vi "kDelay.vi"(8 "delay":i32=10, 11 "input":dbl) -> (3 "output":dbl)   [LabVIEW 2016, in "kevLib2010.lvlib"]
uses:
  kevLib2010.lvlib
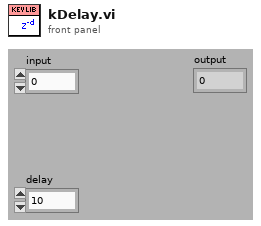
[diagram p1: front panel]
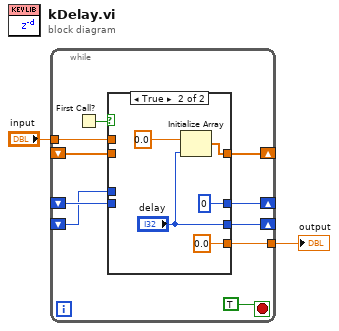
[diagram p0: block diagram]
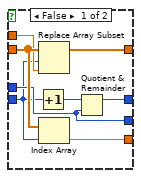
[diagram p2: hidden frame]
diagram:
  n1 = while {
    shift-right: [w11] -> _
    shift-left: _ -> [w10]
    shift-right: [w9] -> _
    shift-left: _ -> [w8]
    shift-right: [w7] -> _
    shift-left: _ -> [w6]
    tunnel: "input" -> [w5]
    tunnel: [w3] -> w1
    stop <- TRUE stop-if-true
    n2 = First Call?() -> (First Call?: T/F=w12:bool)
    n3 = case shown="True" w12 {
      tunnel: [w19 w25] -> w11
      tunnel: w10 -> [w20 _]
      tunnel: [w16 0 ("index")] -> w9
      tunnel: w8 -> [w14 _]
      tunnel: [w17 "delay"] -> w7
      tunnel: w6 -> [w17 _]
      tunnel: w5 -> [w15 _]
      tunnel: [w13 0.0 ("input")] -> w3
      frame False {
        n4 = Increment(x=w14) -> (x+1=w18:i32)
        n5 = Replace Array Subset(array=w20, new element=w15, index=w14) -> (w19:dbl[])
        n6 = Index Array(array=w20, index=w14) -> (element=w13:dbl)
        n7 = Quotient & Remainder(x=w18, y=w17) -> (x-y*floor(x/y)=w16:i32)  [unwired: 1 out]
      }
      frame True {
        n8 = Initialize Array(0.0 ("input"), "delay") -> (w25:dbl[])
      }
    }
  }
  "output" <- w1
